vi "tasklist_read.vi"(8 "error in (no error)":errorcluster) -> (0 "error out":errorcluster, 3 "tasklist":T1)   [LabVIEW 2015, in "lv-bin-windows.lvlib" / "v1.lvlib"]
uses:
  v1.lvlib
  <userlib>/antonio-alexander/lv-bin/lv-bin/public/api/v1/v1.lvlib
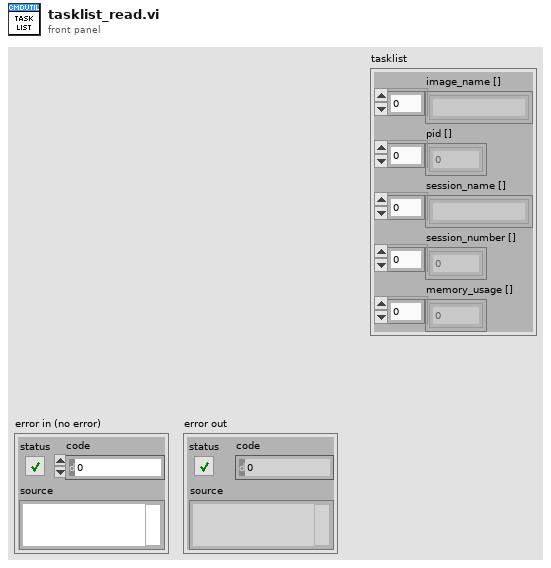
[diagram p1: front panel]
types:
  T1 = cluster{"image_name []":string[], "pid []":i32[], "session_name []":string[], "session_number []":i32[], "memory_usage []":dbl[]}
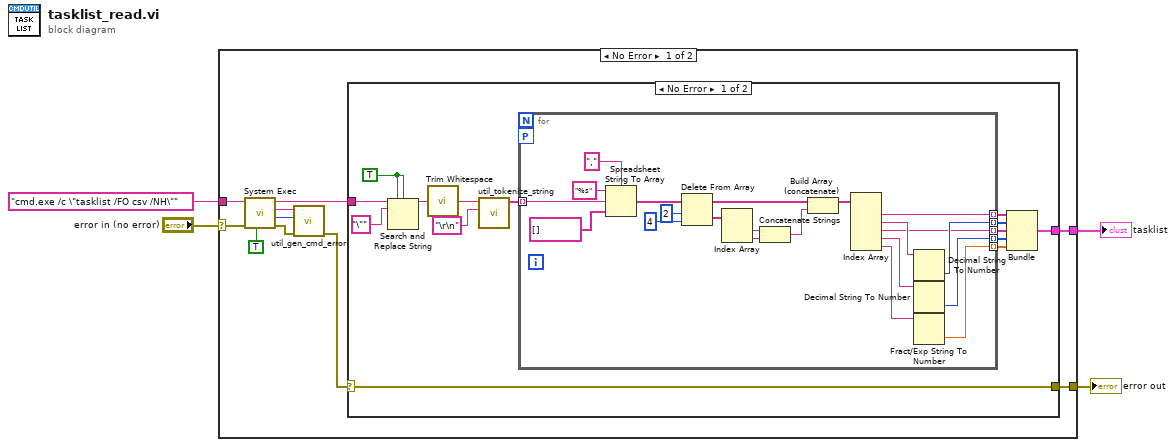
[diagram p0: block diagram]
diagram:
  n1 = case shown="No Error" "error in (no error)" {
    selector: "error in (no error)" -> [w9 w51]
    tunnel: [w10 w51] -> w4
    tunnel: "cmd.exe /c \"tasklist /FO csv /NH\"" ("command line") -> [w8 _]
    tunnel: [w7 _] -> w1
    frame No Error {
      n2 = call <vilib>:"System Exec.vi"("run minimized? (F)"=TRUE, "error in (no error)"=w9, "command line"=w8) -> ("error out"=w13:errorcluster, "return code"=w5:i32, "standard error"=w6:string, "standard output"=w12:string)  [unwired: 5 in]
      n3 = call <userlib>:"util_gen_cmd_error.vi"("error in (no error)"=w13, "return_code"=w5, "standard_error"=w6) -> ("error out"=w11:errorcluster)  [unwired: 8 in]
      n4 = case shown="No Error" w11 {
        selector: w11 -> [w28 w50]
        tunnel: w12 -> [w27 _]
        tunnel: [w28 w50] -> w10
        tunnel: [w15 _] -> w7
        frame No Error {
          w22 = TRUE ("replace all? (F)")
          n5 = Search and Replace String(replace all?=w22, case sensitive?=w22, input string=w27, search string="\"") -> (result string=w24:string)  [unwired: 4 in, 3 out]
          n6 = call <vilib>:"Trim Whitespace.vi"("string"=w24) -> ("trimmed string"=w23:string)  [unwired: 1 in]
          n7 = call <userlib>:"util_tokenize_string.vi"("delimiter"="\r\n", "input_string"=w23) -> ("before_match []"=w26:string[])  [unwired: 7 in, 2 out]
          n8 = for {
            tunnel: w26 -> [w49] mode=indexing
            tunnel: [w33] -> w20 mode=indexing
            tunnel: [w32] -> w19 mode=indexing
            tunnel: [w31] -> w18 mode=indexing
            tunnel: [w30] -> w17 mode=indexing
            tunnel: [w29] -> w16 mode=indexing
            workers-P: _ -> [_]
            n9 = Spreadsheet String To Array(delimiter (Tab)=",", format string="%s", spreadsheet string=w49, array type (2D Dbl)=string[] [] ("array")) -> (array=w44:string[])
            n10 = Delete From Array(array=w44, length=2, index=4) -> (deleted portion=w43:string[], array with subset deleted=w38:string[])
            n11 = Index Array(array=w43) -> (element #1=w42:string, element #2=w40:string)  [unwired: 2 in]
            n12 = Concatenate Strings(w42, w40) -> (w39:string)
            n13 = Build Array (concatenate)(w38, w39) -> (w37:string[])
            n14 = Index Array(array=w37) -> (element #1=w33:string, element #2=w36:string, element #3=w31:string, element #4=w35:string, element #5=w34:string)  [unwired: 5 in]
            n15 = Decimal String To Number(string=w36) -> (number=w32:i32)  [unwired: 2 in, 1 out]
            n16 = Decimal String To Number(string=w35) -> (number=w30:i32)  [unwired: 2 in, 1 out]
            n17 = Fract/Exp String To Number(string=w34) -> (number=w29:dbl)  [unwired: 3 in, 1 out]
          }
          n18 = Bundle(w20, w19, w18, w17, w16) -> (w15:cluster{string[], i32[], string[], i32[], dbl[]})  [unwired: 1 in]
        }
        frame Error {
        }
      }
    }
    frame Error {
    }
  }
  "error out" <- w4
  "tasklist" <- w1
